vi "buildMFCinfoMessage.vi"(11 "DataBus in":T1 {"RhoTrace" format="%.3gg/l"; "RhoCarrier" format="%.3gg/l"; "InactiveC2H6MFCs"."mDot" format="%_4g"; "InactiveC2H6MFCs"."Setpoint" format="%.2g"; "InactiveC2H6MFCs"."MFCcapability"."MaxMdot" format="%_4g"; "InactiveC2H6MFCs"."MFCcapability"."MinMdot" format="%_4g"; "ActiveC2H6MFCs"."mDot" format="%_4g"; "ActiveC2H6MFCs"."Setpoint" format="%.2g"; "ActiveC2H6MFCs"."MFCcapability"."MaxMdot" format="%_4g"; "ActiveC2H6MFCs"."MFCcapability"."MinMdot" format="%_4g"; "InactiveN2MFCs"."mDot" format="%_4g"; "InactiveN2MFCs"."Setpoint" format="%.2g"; "InactiveN2MFCs"."MFCcapability"."MaxMdot" format="%_4g"; "InactiveN2MFCs"."MFCcapability"."MinMdot" format="%_4g"; "ActiveN2MFCs"."mDot" format="%_4g"; "ActiveN2MFCs"."Setpoint" format="%.2g"; "ActiveN2MFCs"."MFCcapability"."MaxMdot" format="%_4g"; "ActiveN2MFCs"."MFCcapability"."MinMdot" format="%_4g"; "C2H6MFCs"."mDot" format="%_4g"; "C2H6MFCs"."Setpoint" format="%.2g"; "C2H6MFCs"."MFCcapability"."MaxMdot" format="%_4g"; "C2H6MFCs"."MFCcapability"."MinMdot" format="%_4g"; "N2MFCs"."mDot" format="%_4g"; "N2MFCs"."Setpoint" format="%.2g"; "N2MFCs"."MFCcapability"."MaxMdot" format="%_4g"; "N2MFCs"."MFCcapability"."MinMdot" format="%_4g"; "QdemCarrier" format="%.2pl/min"; "QdemTrace" format="%.2pl/min"; "MdotCarrier" format="%_4pg/min"; "MdotTrace" format="%_4pg/min"; "releaseTemp" format="%#_gC"; "releasePress" format="%#_gmBar"}) -> (3 "infoString":string)   [LabVIEW 2016]
uses:
  AalborgServerData.ctl
  MFCdescription.ctl
  MFCcapability.ctl
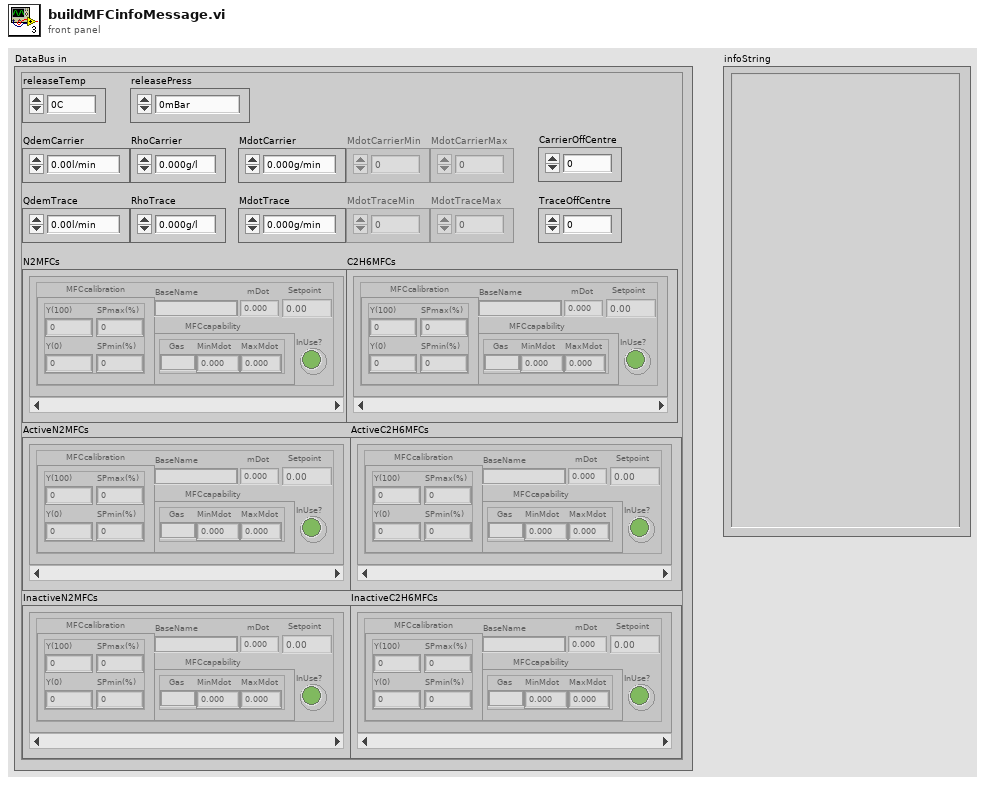
[diagram p1: front panel]
types:
  T1 = typedef "AalborgServerData.ctl" = cluster{"releaseTemp":dbl, "releasePress":dbl, "QdemCarrier":dbl, "QdemTrace":dbl, "MdotCarrier":dbl, "MdotCarrierMin":dbl, "MdotCarrierMax":dbl, "MdotTrace":dbl, "MdotTraceMin":dbl, "MdotTraceMax":dbl, "N2MFCs":T2[], "C2H6MFCs":T2[], "CarrierOffCentre":dbl, "TraceOffCentre":dbl, "ActiveN2MFCs":T2[], "InactiveN2MFCs":T2[], "ActiveC2H6MFCs":T2[], "InactiveC2H6MFCs":T2[], "RhoCarrier":dbl, "RhoTrace":dbl}
  T2 = typedef "MFCdescription.ctl" = cluster{"BaseName":string, "MFCcalibration":cluster{"Y(100)":dbl, "Y(0)":dbl, "SPmin(%)":dbl, "SPmax(%)":dbl}, "MFCcapability":T3, "InUse?":bool, "Setpoint":dbl, "mDot":dbl}
  T3 = typedef "MFCcapability.ctl" = cluster{"Gas":string, "MinMdot":dbl, "MaxMdot":dbl}
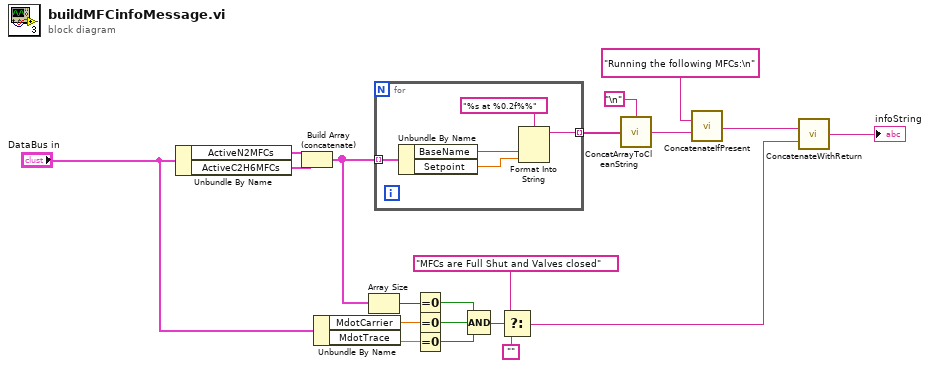
[diagram p0: block diagram]
diagram:
  n1 = Unbundle By Name("DataBus in") -> ("ActiveN2MFCs"=w12:T2[], "ActiveC2H6MFCs"=w19:T2[])
  n2 = Build Array (concatenate)(w12, w19) -> (w11:T2[])
  n3 = Unbundle By Name("DataBus in") -> ("MdotCarrier"=w14:dbl, "MdotTrace"=w13:dbl)
  n4 = Array Size(array=w11) -> (size(s)=w10:i32)
  n5 = for {
    tunnel: w11 -> [w25] mode=indexing
    tunnel: [w21] -> w20 mode=indexing
    n6 = Unbundle By Name(w25) -> ("BaseName"=w24:string, "Setpoint"=w23:dbl)
    n7 = Format Into String(format string="%s at %0.2f%%", w24, w23) -> (resulting string=w21:string)  [unwired: 2 in, 1 out]
  }
  n8 = Equal To 0?(x=w10) -> (x = 0?=w9:bool)
  n9 = Equal To 0?(x=w14) -> (x = 0?=w7:bool)
  n10 = Equal To 0?(x=w13) -> (x = 0?=w8:bool)
  n11 = Compound Arithmetic op=AND(w9, w7, w8) -> (w6:bool)
  n12 = Select(t="MFCs are Full Shut and Valves closed" ("string"), s=w6, f="") -> (s? t:f=w1:string)
  n13 = call "ConcatArrayToCleanString.vi"("stringArray"=w20, "separator(;)"="\n") -> ("cleanDelimitedString"=w17:string)
  n14 = call "ConcatenateIfPresent.vi"("prependString"="Running the following MFCs:\n" ("string"), "appendString"=w17) -> ("outputString"=w3:string)  [unwired: 13 in]
  n15 = call "ConcatenateWithReturn.vi"("baseString"=w3, "additionalString"=w1) -> ("outputString"=→"infoString":string)  [unwired: 13 in]
